vi "insertFT_USE.vi"(0 "M100 Monitor Board":string[][](table), 1 "connection reference":T1, 3 "error in (no error)":errorcluster) -> (7 "connection reference out":T1, 10 "error out":errorcluster)   [LabVIEW 2012]
uses:
  <vilib>/addons/database/Connection.llb/Conn ObjectReference.ctl
  <vilib>/addons/database/NI_Database_API.lvlib
panel:
  out "trimmed string":string
  in  "Cluster":T2
  # "p"
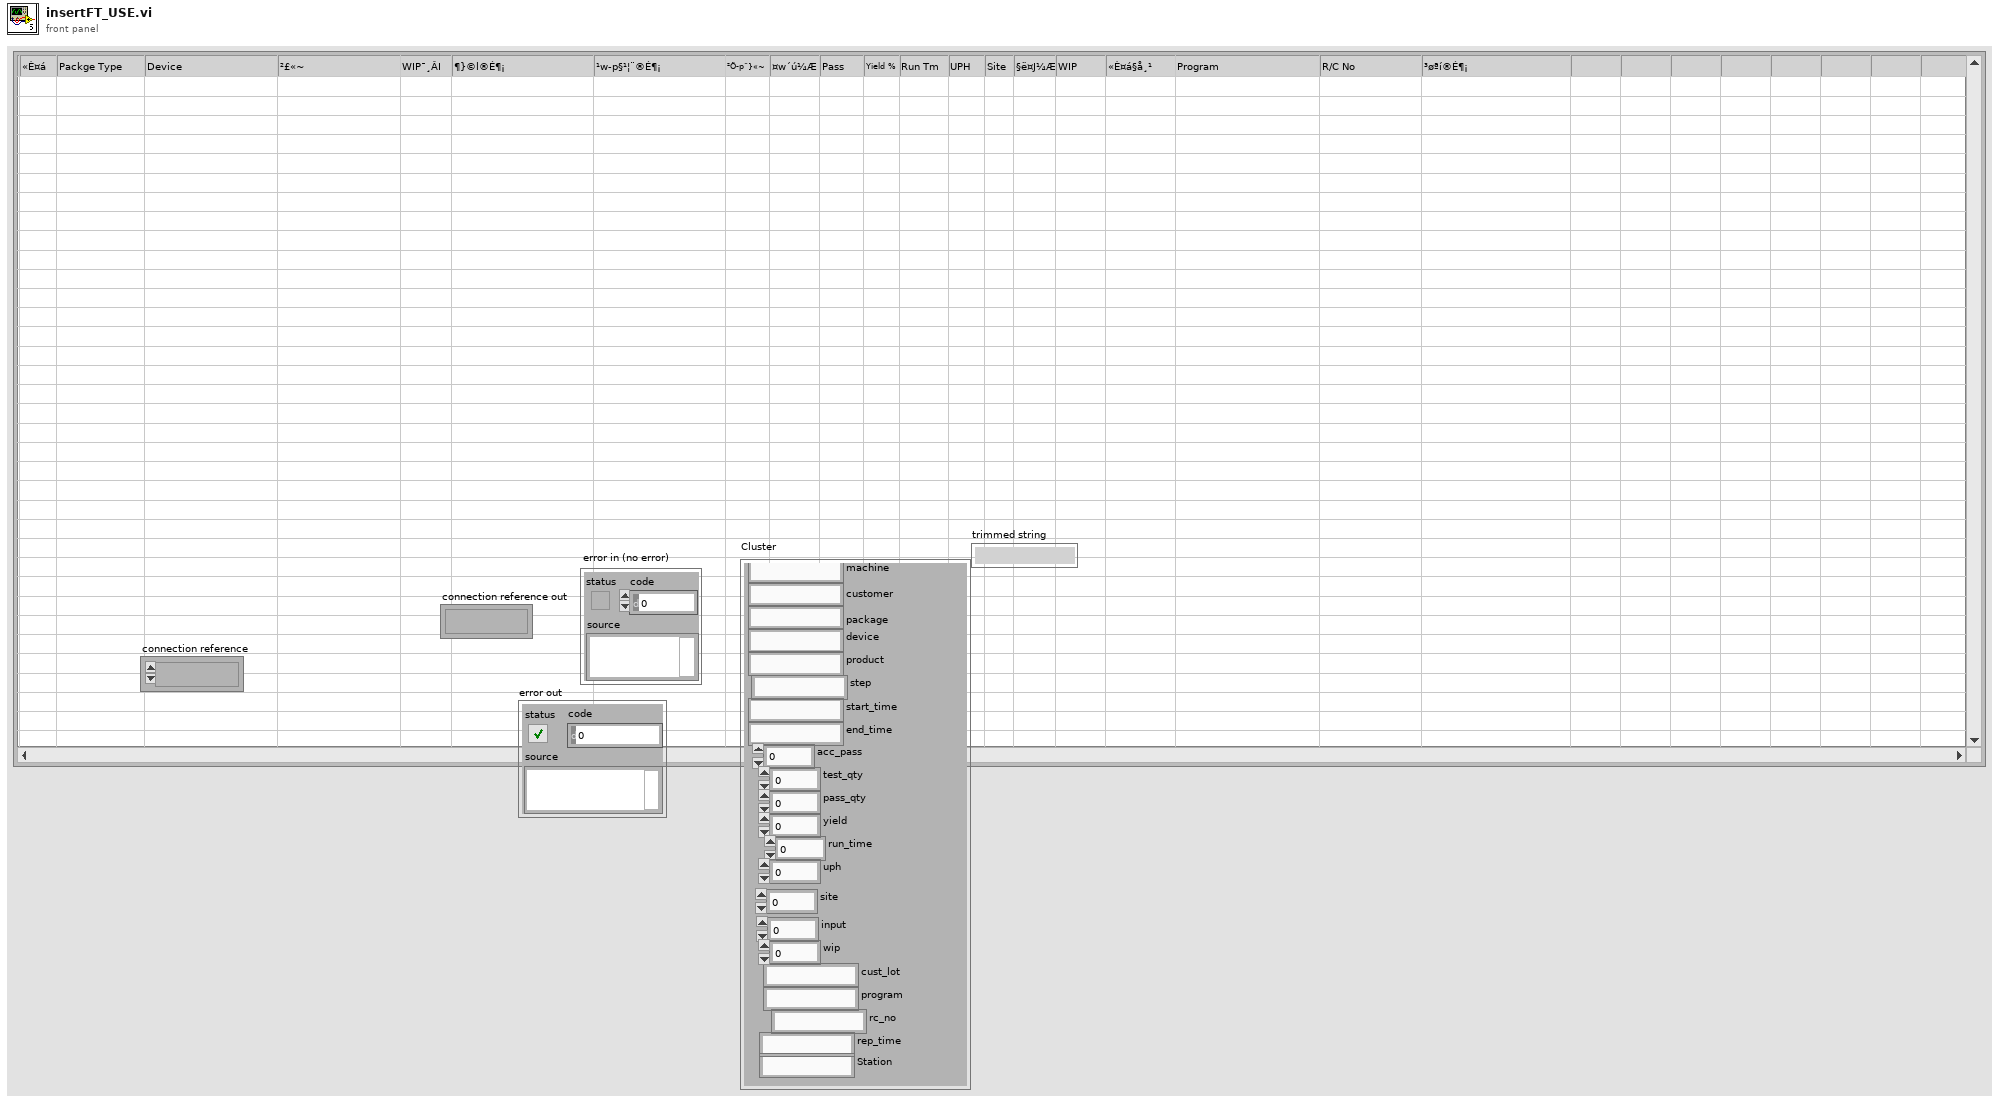
[diagram p1: front panel]
types:
  T1 = typedef "NI_Database_API.lvlib/Conn ObjectReference.ctl" = refnum<k1>
  T2 = cluster{"machine":string, "customer":string, "package":string, "device":string, "product":string, "step":string, "start_time":string, "end_time":string, "acc_pass":dbl, "test_qty":dbl, "pass_qty":dbl, "yield":dbl, "run_time":dbl, "uph":dbl, "site":dbl, "input":dbl, "wip":dbl, "cust_lot":string, "program":string, "rc_no":string, "rep_time":string, "Station":string}
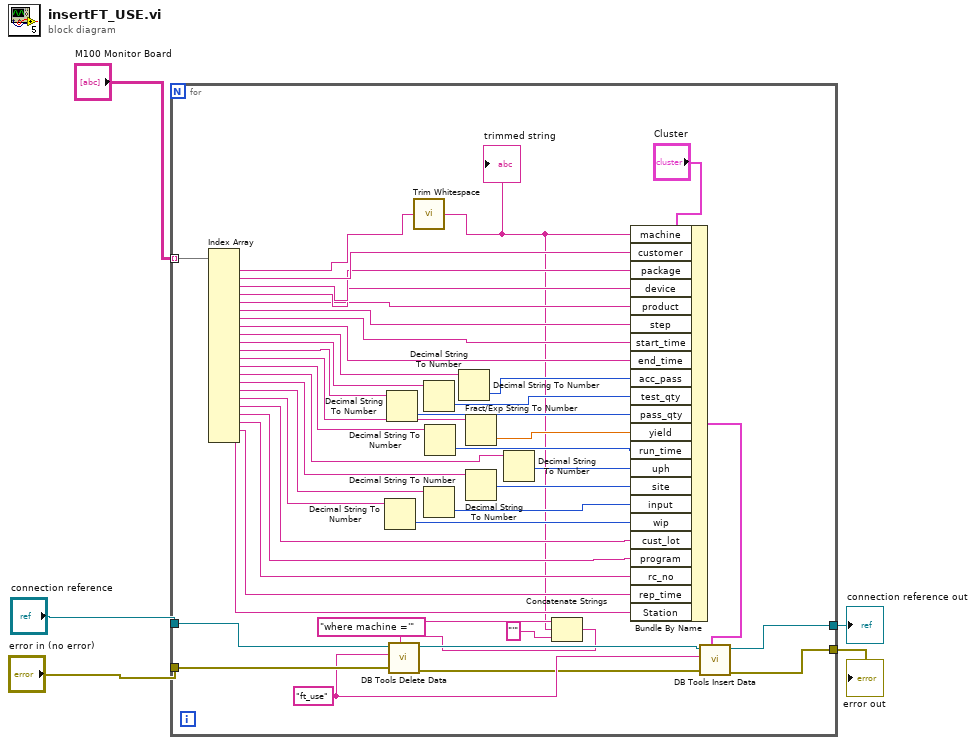
[diagram p0: block diagram]
diagram:
  n1 = for {
    tunnel: "M100 Monitor Board" -> [w50] mode=indexing
    tunnel: "connection reference" -> [w14]
    tunnel: "error in (no error)" -> [w15]
    tunnel: [w19] -> w4
    tunnel: [w18] -> w1
    w13 = "ft_use" ("table")
    n2 = Index Array(array=w50) -> (element #1=w7:string, element #2=w49:string, element #3=w48:string, element #4=w47:string, element #5=w45:string, element #6=w44:string, element #7=w43:string, element #8=w42:string, element #9=w41:string, element #10=w38:string, element #11=w37:string, element #12=w34:string, element #13=w33:string, element #14=w27:string, element #15=w26:string, element #16=w25:string, element #17=w24:string, element #18=w23:string, element #19=w22:string, element #20=w21:string, element #21=w20:string, element #22=w16:string)  [unwired: 22 in]
    n3 = Decimal String To Number(string=w24) -> (number=w32:i32)  [unwired: 2 in, 1 out]
    n4 = Decimal String To Number(string=w37) -> (number=w36:i32)  [unwired: 2 in, 1 out]
    n5 = call <vilib>:"Trim Whitespace.vi"("string"=w7) -> ("trimmed string"=w6:string)  [unwired: 1 in]
    "trimmed string" <- w6
    n6 = Decimal String To Number(string=w38) -> (number=w39:i32)  [unwired: 2 in, 1 out]
    n7 = Decimal String To Number(string=w25) -> (number=w31:i32)  [unwired: 2 in, 1 out]
    n8 = Decimal String To Number(string=w33) -> (number=w28:i32)  [unwired: 2 in, 1 out]
    n9 = Decimal String To Number(string=w41) -> (number=w40:i32)  [unwired: 2 in, 1 out]
    n10 = Fract/Exp String To Number(string=w34) -> (number=w35:dbl)  [unwired: 3 in, 1 out]
    n11 = Decimal String To Number(string=w26) -> (number=w30:i32)  [unwired: 2 in, 1 out]
    n12 = Decimal String To Number(string=w27) -> (number=w29:i32)  [unwired: 2 in, 1 out]
    n13 = Concatenate Strings("where machine ='" ("condition"), w6, "'" ("string")) -> (w8:string)
    n14 = call <vilib>:"DB Tools Delete Data.vi"("condition"=w8, "error in (no error)"=w15, "table"=w13, "connection reference"=w14) -> ("error out"=w11:errorcluster, "connection reference out"=w12:T1)  [unwired: 6 in]
    n15 = Bundle By Name(cluster="Cluster", "machine"=w6, "customer"=w49, "package"=w48, "device"=w47, "product"=w45, "step"=w44, "start_time"=w43, "end_time"=w42, "acc_pass"=w40, "test_qty"=w39, "pass_qty"=w36, "yield"=w35, "run_time"=w28, "uph"=w29, "site"=w30, "input"=w31, "wip"=w32, "cust_lot"=w23, "program"=w22, "rc_no"=w21, "rep_time"=w20, "Station"=w16) -> (w17:T2)
    n16 = call <vilib>:"DB Tools Insert Data.vi"("data"=w17, "error in (no error)"=w11, "table"=w13, "connection reference"=w12) -> ("error out"=w18:errorcluster, "connection reference out"=w19:T1)  [unwired: 6 in]
  }
  "connection reference out" <- w4
  "error out" <- w1
